vi "S2020_GSW.vi"() -> ()   [LabVIEW 2020]
uses:
  Subs/Server XCtrl/Server.xctl
  <vilib>/Platform/browser.llb/Open URL in Default Browser (string).vi
panel:
  in  "Tab Control":enum32{"MicroPython", "LabVIEW", "TensorFlow"}(tab)
  in  "Useful VIs":bool
  in  "IDE":bool
  in  "Docs":bool
  in  "New VI":bool
  in  "Server":path(xcontrol)=path "/Users/crogers/GitHub/Summer2020/LabVIEWCode/Servers/Jens.vi"
  in  "Help":bool
  in  "Open Server":bool
  in  "Simple Comm":bool
  in  "Examples":i32(listbox)
  out "Diagram":picture
  in  "YouTube":bool
  in  "TensorFlow":bool
  # "Summer\n2020"
  # "Train your machine at https://teachablemachine.withgoogle.com"
  # "Make sure you \n1. have Python 3.7 on your machine and 64/32 bit like your LabVIEW (with an updated pip)\n2. pip3.7 install tensorflow   (for AI) https://www.tensorflow.org/install/pip\n3. pip3.7 install opencv-python   (for image processing)  https://pypi.org/project/opencv-python/\n4. pip3.7 install paramiko  (for SSH talking to the EV3) http://www.paramiko.org/installing.html\n5. pip3.7 install scp"
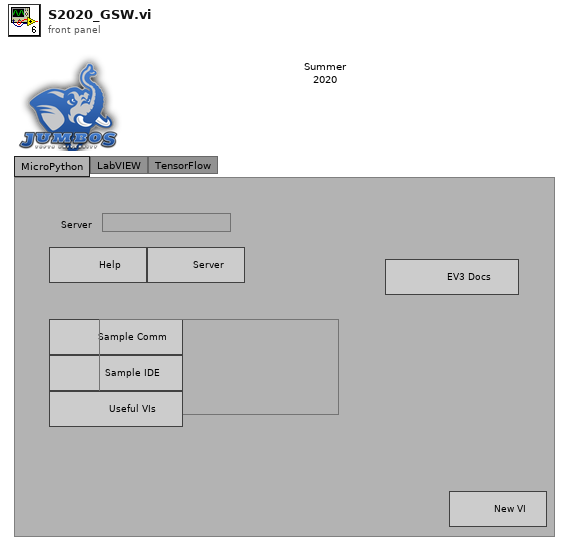
[diagram p1: front panel]
types:
  T1 = enum32{"Invalid", "Standard", "Closed", "Hidden", "Minimized", "Maximized"}
  T2 = typedef "LVBoundsTypeDef.ctl" = cluster{"Width":u32, "Height":u32}
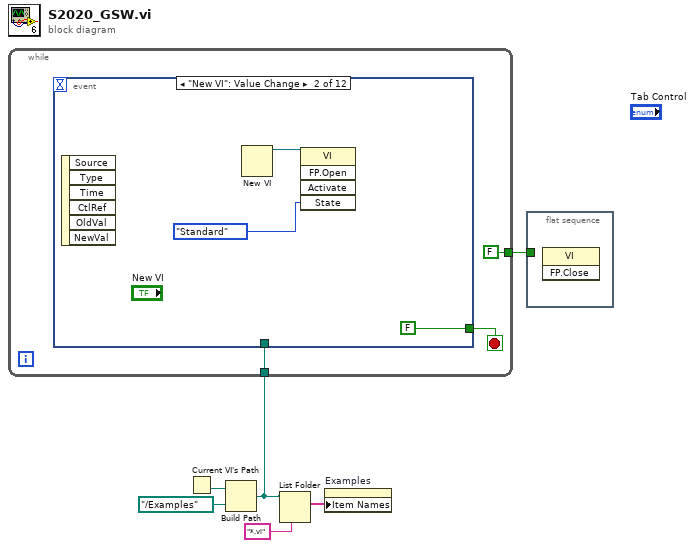
[diagram p0: block diagram]
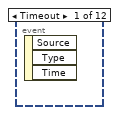
[diagram p2: hidden frame]
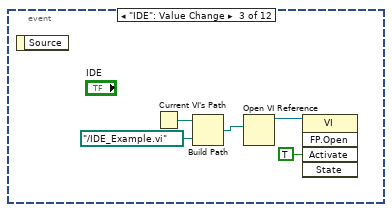
[diagram p3: hidden frame]
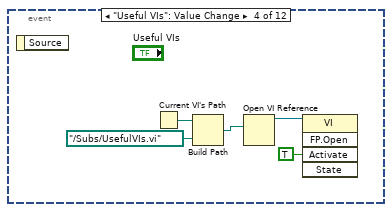
[diagram p4: hidden frame]
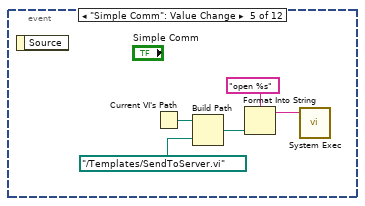
[diagram p5: hidden frame]
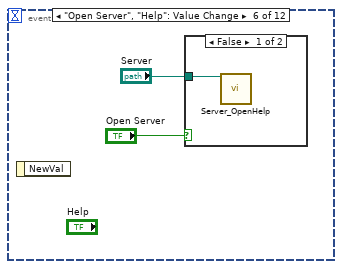
[diagram p6: hidden frame]
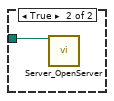
[diagram p7: hidden frame]
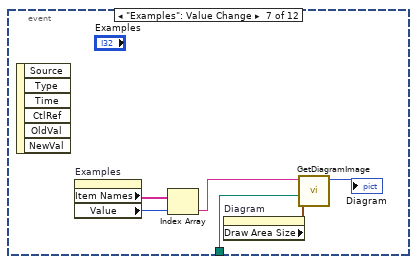
[diagram p8: hidden frame]
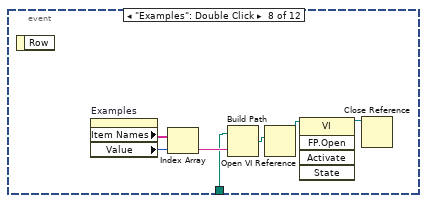
[diagram p9: hidden frame]
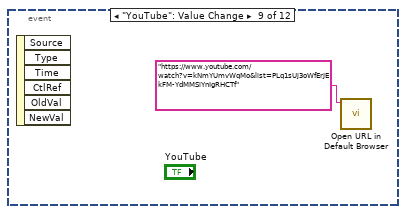
[diagram p10: hidden frame]
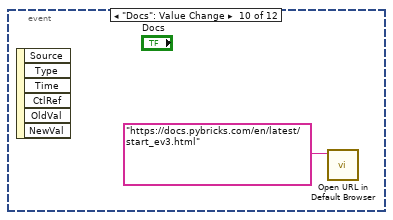
[diagram p11: hidden frame]
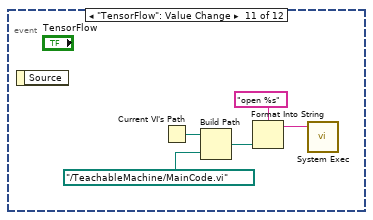
[diagram p12: hidden frame]
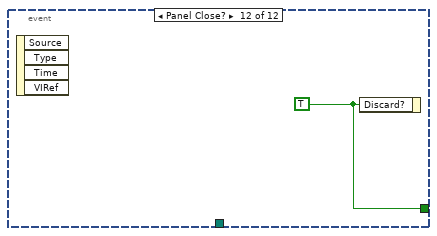
[diagram p13: hidden frame]
diagram:
  n1 = Current VI's Path() -> (path=w4:path)
  n2 = Build Path(base path=w4, name or relative path=path "../Examples") -> (appended path=w2:path)
  n3 = while {
    tunnel: [FALSE] -> w6
    tunnel: w2 -> [w7]
    stop <- w9 stop-if-true
    n4 = event shown="[1] \"New VI\": Value Change" {
      selector: _ -> [_ _ _ _ _ _ _ _ _ _ _ _]
      dyn-events: _ -> [_ _ _ _ _ _ _ _ _ _ _ _]
      timeout: _ -> [_ _ _ _ _ _ _ _ _ _ _ _]
      tunnel: [_ FALSE ("Discard?") _ _ _ _ _ _ _ _ _ w52] -> w9
      tunnel: w7 -> [_ _ _ _ _ _ w34 w38 _ _ _ _]
      event Timeout {
        n5 = event-data() -> ()  [unwired: 1 in, 3 out]
      }
      event "New VI": Value Change {
        n6 = event-data() -> ()  [unwired: 1 in, 6 out]
        n7 = New VI() -> (3:w11:refnum<vi>)  [unwired: 7 in, 1 out]
        n8 = invoke class="VI" method="FP.Open"(reference=w11, "State"=T1."Standard") -> ()  [unwired: 3 in, 5 out]
      }
      event "IDE": Value Change {
        n9 = event-data() -> ()  [unwired: 1 in, 1 out]
        n10 = Current VI's Path() -> (path=w17:path)
        n11 = Build Path(base path=w17, name or relative path=path "../IDE_Example.vi") -> (appended path=w15:path)
        n12 = Open VI Reference(vi path=w15) -> (vi reference=w14:refnum<vi>)  [unwired: 5 in, 1 out]
        n13 = invoke class="VI" method="FP.Open"(reference=w14, "Activate"=TRUE ("Activate?")) -> ()  [unwired: 3 in, 5 out]
      }
      event "Useful VIs": Value Change {
        n14 = event-data() -> ()  [unwired: 1 in, 1 out]
        n15 = Current VI's Path() -> (path=w22:path)
        n16 = Build Path(base path=w22, name or relative path=path "../Subs/UsefulVIs.vi") -> (appended path=w20:path)
        n17 = Open VI Reference(vi path=w20) -> (vi reference=w19:refnum<vi>)  [unwired: 5 in, 1 out]
        n18 = invoke class="VI" method="FP.Open"(reference=w19, "Activate"=TRUE ("Activate?")) -> ()  [unwired: 3 in, 5 out]
      }
      event "Simple Comm": Value Change {
        n19 = event-data() -> ()  [unwired: 1 in, 1 out]
        n20 = Current VI's Path() -> (path=w27:path)
        n21 = Build Path(base path=w27, name or relative path=path "../Templates/SendToServer.vi") -> (appended path=w23:path)
        n22 = Format Into String(format string="open %s", w23) -> (resulting string=w25:string)  [unwired: 2 in, 1 out]
        n23 = call <vilib>:"System Exec.vi"("command line"=w25) -> ()  [unwired: 7 in, 4 out]
      }
      event "Open Server", "Help": Value Change {
        n24 = event-data() -> ()  [unwired: 1 in, 1 out]
        n25 = case shown="False" "Open Server" {
          tunnel: "Server" -> [w30 w31]
          frame False {
            n26 = call "Server_OpenHelp.vi"("Server"=w30) -> ()  [unwired: 10 in, 1 out]
          }
          frame True {
            n27 = call "Server_OpenServer.vi"("Server"=w31) -> ()  [unwired: 10 in, 1 out]
          }
        }
      }
      event "Examples": Value Change {
        n28 = event-data() -> ()  [unwired: 1 in, 6 out]
        n29 = property on="Examples" class="LstBox (strict)"() -> ("Item Names"=w37:string[], "Value"=w36:i32)  [unwired: 2 in, 2 out]
        n30 = Index Array(array=w37, index=w36) -> (element=w35:string)
        n31 = property on="Diagram" class="Pict"() -> ("Draw Area Size"=w33:T2)  [unwired: 2 in, 2 out]
        n32 = call "GetDiagramImage.vi"("Draw Area Size"=w33, "appended path"=w34, "String"=w35) -> ("2D Picture"=→"Diagram":picture)  [unwired: 8 in]
      }
      event "Examples": Double Click {
        n33 = event-data() -> ()  [unwired: 1 in, 1 out]
        n34 = property on="Examples" class="LstBox (strict)"() -> ("Item Names"=w44:string[], "Value"=w43:i32)  [unwired: 2 in, 2 out]
        n35 = Index Array(array=w44, index=w43) -> (element=w39:string)
        n36 = Build Path(base path=w38, name or relative path=w39) -> (appended path=w40:path)
        n37 = Open VI Reference(vi path=w40) -> (vi reference=w41:refnum<vi>)  [unwired: 5 in, 1 out]
        n38 = invoke class="VI" method="FP.Open"(reference=w41) -> (reference out=w42:refnum<vi>)  [unwired: 4 in, 4 out]
        n39 = Close Reference(reference=w42) -> ()  [unwired: 1 in, 1 out]
      }
      event "YouTube": Value Change {
        n40 = event-data() -> ()  [unwired: 1 in, 6 out]
        n41 = call-poly <vilib>:"Open URL in Default Browser.vi"("URL"="https://www.youtube.com/watch?v=kNmYUmvWqMo&list=PLq1sUj3oWfErJEkFM-YdMMSiYnIgRHCTf") -> ()  [unwired: 5 in, 2 out]
      }
      event "Docs": Value Change {
        n42 = event-data() -> ()  [unwired: 1 in, 6 out]
        n43 = call-poly <vilib>:"Open URL in Default Browser.vi"("URL"="https://docs.pybricks.com/en/latest/start_ev3.html") -> ()  [unwired: 5 in, 2 out]
      }
      event "TensorFlow": Value Change {
        n44 = event-data() -> ()  [unwired: 1 in, 1 out]
        n45 = Current VI's Path() -> (path=w51:path)
        n46 = Build Path(base path=w51, name or relative path=path "../TeachableMachine/MainCode.vi") -> (appended path=w47:path)
        n47 = Format Into String(format string="open %s", w47) -> (resulting string=w49:string)  [unwired: 2 in, 1 out]
        n48 = call <vilib>:"System Exec.vi"("command line"=w49) -> ()  [unwired: 7 in, 4 out]
      }
      event Panel Close? {
        w52 = TRUE ("Discard?")
        n49 = event-data() -> ()  [unwired: 1 in, 4 out]
        n50 = event-data("Discard?"=w52) -> ()  [unwired: 1 in, 1 out]
      }
    }
  }
  n51 = List Folder(path=w2, pattern="*.vi") -> (filenames=w3:string[])  [unwired: 2 in, 3 out]
  n52 = property on="Examples" class="LstBox (strict)"("Item Names"=w3) -> ()  [unwired: 2 in, 2 out]
  n53 = flat-sequence {
    tunnel: w6 -> [_]
    frame #0 {
      n54 = invoke class="VI" method="FP.Close"() -> ()  [unwired: 3 in, 3 out]
    }
  }
